vi "New Marker.vi"() -> (2 "Longitude":string, 3 "Latitude":string)   [LabVIEW 2012]
panel:
  in  "Ok":bool
  in  "Longitude":dbl
  in  "Latitude":dbl
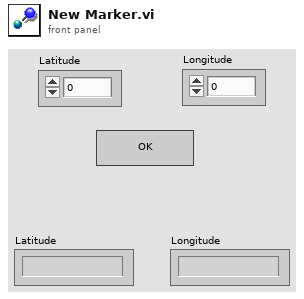
[diagram p1: front panel]
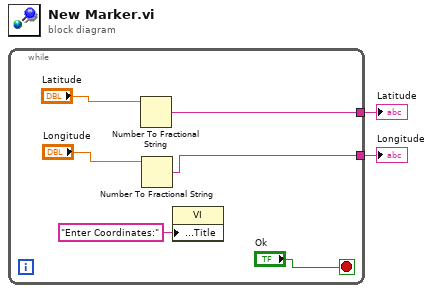
[diagram p0: block diagram]
diagram:
  n1 = while {
    tunnel: [w5] -> w2
    tunnel: [w4] -> w1
    stop <- "Ok" stop-if-true
    n2 = Number To Fractional String(number="Latitude") -> (F-format string=w5:string)  [unwired: 3 in]
    n3 = Number To Fractional String(number="Longitude") -> (F-format string=w4:string)  [unwired: 3 in]
    n4 = property class="VI"("Front Panel.Title"="Enter Coordinates:" ("Front Panel Window:Title")) -> ()  [unwired: 2 in, 2 out]
  }
  "Latitude" <- w2
  "Longitude" <- w1
